vi "21_1.vi"() -> ()   [LabVIEW 2020]
uses:
  <userlib>/_OpenG.lib/array/array.llb/Remove Duplicates from 1D Array (String)__ogtk.vi
  <userlib>/_OpenG.lib/array/array.llb/Index 1D Array Elements (String)__ogtk.vi
panel:
  out "size(s)":i32=1679
  out "Array":string[](array[string])=["tksps", "nmzblnq", "pzz", "gkmdkp", "fdpp", "htdps", "njvzpr", "lsfn", "vxbnd", "qvft", "nmpt", "ptq", "dckbmh", "bh", "xxlb", "pbjp", "zlpbptr", "mmphj", "ddc", "zxmkkpp", "jrgrcz", "xzhmdb", "mqkf", "bmcj", "lsv", "bsbz", "mklt", "nkmj", "crbt", "zxcqtf", "rjbsr", "hbcgjtx", "vvqpqgl", "rnbfzg", "hxndkq", "vrntfjx", "clmk", "zdslsk", "ljczhn", "fkntrq", "kbkkrlfq", "bt", "mrz", "nhpsk", "lsc", "vqjj", "lfd", "bsllxjtm", "zdpcb", "qpjplfl", "gkcskhp", "vrbxt", "ftnhrx", "fbjbkp", "sffzz", "pzvvt", "phth", "mlftm", "kbkkrlfq", "dtqq", "jdnlg", "dlxp", "ljczhn", "zrngn", "qnlrbn", "lbxc", "chjdk", "fkntrq", "xxlb", "pcvh", "xmgc", "vkzh", "pzz", "sgv", "xlc", "xmjr", "bqtpqsp", "vrntfjx", "xxx", "xzhmdb", "vpsd", "clptg", "qpjplfl", "fcrvj", "nmzblnq", "cxgmp", "jqcfq", "sbr", "xbdmll", "jtknrjp", "fcdtf", "bbxvmgs", "mgjdd", "dckbmh", "ns", "fdpp", "pbjp", "xbtpfxjz", "fbvdlb", "mrz", "ftnhrx", "fsddds", "hsmkqgx", "gkmdkp", "xxdmj", "cksrd", "zgbbl", "zdslsk", "zpqbb", "bgkf", "rnbfzg", "bhgzdg", "ndmjr", "nhpsk", "fjndll", "cfnc", "pmqmmxs", "rqpd", "mqkf", "snpxpkvj", "bh", "zbsqdm", "lxkbkkx", "lcpcmk", "xbdmll", "ttszmr", "pzvvt", "jbhhjx", "qfqnpf", "dckbmh", "zgbbl", "vrbxt", "dzbxmn", "bsllxjtm", "dblf", "mlftm", "htdps", "ldprd", "tllqrt", "sfprzmk", "zrngn", "lmxfpn", "hxndkq", "gkcskhp", "bqtpqsp", "chjdk", "kzfsztx", "nkmj", "tjxxdmq", "ztlp", "vvzf", "vplt", "bhgzdg", "gsshb", "bmjx", "fjndll", "clmk", "qbrgtl", "ndmjr", "xzhmdb", "bpzlm", "kspf", "gvhrgz", "ddcrr", "fdpp", "tlgbjhs", "xvqmjsc", "lsc", "mqkf", "lsv", "krrsrp", "zsbzn", "bkxnht", "mgjdd", "jbtjxtf", "slbrp", "kchnq", "vpsd", "zdpcb", "ftnhrx", "sm", "mcdsfh", "xplxv", "fkntrq", "gntk", "tksps", "sbr", "vbxdp", "vtdd", "lrbpxs", "dgnrq", "ktm", "xlc", "jrgrcz", "lkdrpt", "rqpd", "xgzbl", "fjndll", "ddcrr", "xbhsqv", "pqjgdkl", "lxkbkkx", "kttchg", "vvzf", "xxdmj", "xzhmdb", "pbjp", "fcdtf", "kbkkrlfq", "bpzlm", "qlbxr", "ptq", "kzfsztx", "dgnrq", "jbhhjx", "vqjj", "qnlrbn", "kckgz", "cnmm", "zgbbl", "lrbpxs", "ztlp", "hnlcp", "zhlgsj", "bgkf", "zdpcb", "xbtpfxjz", "bsllxjtm", "krrsrp", "pzz", "nhpsk", "mrz", "ndmjr", "zmqvhh", "xxlb", "bqtpqsp", "zsbzn", "qlgb", "ztlp", "gvhrgz", "sfprzmk", "vcvmq", "xxlb", "lmxfpn", "njrdhq", "lcpcmk", "ttszmr", "qbrgtl", "tnzvgg", "hbfmpsg", "hshl", "vvqpqgl", "pzz", "dckbmh", "zlpbptr", "slbrp", "xgxk", "qlbxr", "bmcj", "bqtpqsp", "hsmkqgx", "ftnhrx", "qmxfh", "lbnr", "hbcgjtx", "krrsrp", "nmpt", "fxznf", "zpqbb", "vbxdp", "dtqq", "zdslsk", "mgjdd", "vtdd", "kttchg", "rdtkzbf", "qfqnpf", "ndmjr", "zrngn", "ttszmr", "bqtpqsp", "qvft", "nhpsk", "qfqnpf", "pcvh", "qmxfh", "cksrd", "xxlb", "mcdsfh", "bhgzdg", "nklz", "fcdtf", "mqkf", "pkzjrp", "phth", "zpqbb", "xvqmjsc", "pbjp", "dlxp", "fcrvj", "sfprzmk", "hnlcp", "xbtpfxjz", "hxndkq", "gkmdkp", "vxbnd", "pzz", "clptg", "mlftm", "nmzblnq", "pmqmmxs", "cpjsfp", "cfnc", "xmjr", "nmpt", "sbr", "vvqpqgl", "fxznf", "mcrxr", "hgvszq", "ftnhrx", "vpsd", "vqjj", "bsbz", "pmvs", "gntk", "bt", "kckgz", "fzpcbck", "ddc", "tjxxdmq", "vjpcxq", "prjcx", "pzvvt", "mgjdd", "njrdhq", "xxx", "sffzz", "cksrd", "gvhrgz", "nkmj", "xvqmjsc", "jglfn", "cxgmp", "fkntrq", "vxbnd", "bkdpdr", "ddcrr", "hxndkq", "jclqn", "mrz", "vrntfjx", "fbjbkp", "nmpt", "slbrp", "mcrxr", "tnzvgg", "krrsrp", "jtknrjp", "hsmkqgx", "pmqmmxs", "xxlb", "pbjp", "ndmjr", "xlc", "sbr", "gxnxkkh", "bsd", "kzfsztx", "vvzf", "qmxfh", "jrmj", "tksps", "kchnq", "dgnrq", "nmfd", "mcdsfh", "zmqvhh", "bcv", "qvft", "gsshb", "kspf", "lsfn", "zxmkkpp", "pqjgdkl", "tlgbjhs", "hgvszq", "xbhsqv", "rqpd", "xmgc", "kfghxt", "tjxxdmq", "bmcj", "rjbsr", "fmfj", "zhlgsj", "zsbzn", "xmjr", "ktm", "fcrvj", "pzvvt", "vbxdp", "zpqbb", "pkzjrp", "fcdtf", "ddc", "crbt", "kckgz", "dmrxd", "pmsjc", "nmzblnq", "phth", "qpjplfl", "fsddds", "vplt", "bsbz", "vplt", "nkmj", "bmjx", "vvzf", "rdtkzbf", "qpjplfl", "tlgbjhs", "hsmkqgx", "mgjdd", "bsd", "mklt", "xmjr", "xxdmj", "bkdpdr", "fbjbkp", "ktm", "crbt", "vpsd", "pzz", "fzpcbck", "krrsrp", "zpqbb", "cvrqg", "vcvmq", "xxlb", "vtdd", "htdps", "vvqpqgl", "lsv", "clptg", "kttchg", "jbtjxtf", "ljczhn", "vjpcxq", "dblf", "sfprzmk", "bqtpqsp", "dgnrq", "fcdtf", "dzbxmn", "pzvvt", "chjdk", "jtknrjp", "vf", "ptq", "ddcrr", "lsc", "njvzpr", "jrgrcz", "gkmdkp", "nklz", "lsfn", "ttszmr", "jrmj", "mqkf", "jglfn", "jdnlg", "pmvs", "dtqq", "bsd", "jbtjxtf", "njvzpr", "dblf", "hqvv", "bkxnht", "dzjjxr", "xbtpfxjz", "fxznf", "cvrqg", "qpjplfl", "kspf", "fcdtf", "hbcgjtx", "lsfn", "zhlgsj", "dmrxd", "lsc", "lkdrpt", "nmpt", "dlxp", "hshl", "jclqn", "fkntrq", "sffzz", "lxkbkkx", "lsv", "mcrxr", "mgjdd", "bt", "zxcqtf", "zgbbl", "bh", "pthjxs", "htdps", "pkzjrp", "fbjbkp", "vbxdp", "kbkkrlfq", "pmvs", "pcvh", "zdpcb", "ns", "vrntfjx", "zdpcb", "vbxdp", "jbtjxtf", "zhlgsj", "xbdmll", "qlbxr", "xmjr", "qpjplfl", "pqjgdkl", "gsshb", "fkntrq", "mcdsfh", "ddcrr", "bt", "fbvdlb", "jqcfq", "bgkf", "dtqq", "fmfj", "ddc", "bsllxjtm", "kbkkrlfq", "cpjsfp", "jbhhjx", "qlgb", "vrbxt", "fbjbkp", "gntk", "zrngn", "kckgz", "zlpbptr", "qvft", "hnlcp", "lrbpxs", "bkxnht", "cksrd", "vqjj", "sgv", "dmrxd", "slbrp", "rkzkd", "pthjxs", "cvrqg", "fcrvj", "vtdd", "kchnq", "qbrgtl", "mlftm", "fdpp", "zmqvhh", "jrgrcz", "pzz", "kttchg", "xvqmjsc", "pcvh", "ttszmr", "pzvvt", "bmjx", "gkcskhp", "gvhrgz", "cnmm", "krrsrp", "kbkkrlfq", "gsshb", "vbxdp", "sgv", "kzfsztx", "zbsqdm", "kttchg", "gvhrgz", "rkzkd", "jtknrjp", "hsmkqgx", "rjbsr", "hbcgjtx", "bsllxjtm", "dmrxd", "dzbxmn", "jglfn", "vpsd", "tsnzbdtb", "vcvmq", "xxx", "zlpbptr", "fbjbkp", "lbnr", "hnlcp", "mcrxr", "tllqrt", "lsc", "fjndll", "bbxvmgs", "tksps", "bmjx", "xmjr", "mlftm", "qlgb", "ljczhn", "tjxxdmq", "mrz", "kttchg", "pzz", "xmjr", "vvzf", "ktm", "zhlgsj", "zsbzn", "dckbmh", "vcvmq", "jglfn", "zxmkkpp", "fxznf", "xmgc", "hgvszq", "zlpbptr", "hbfmpsg", "tsnzbdtb", "lkdrpt", "vbxdp", "pqjgdkl", "mlftm", "nhpsk", "ptq", "vjpcxq", "gsshb", "cfnc", "ddcrr", "kckgz", "bh", "kzfsztx", "tnzvgg", "dblf", "xbdmll", "vkzh", "pmqmmxs", "vplt", "nklz", "xplxv", "gvhrgz", "lsfn", "jclqn", "lxkbkkx", "prjcx", "mklt", "hsmkqgx", "vtdd", "sm", "vrntfjx", "rjbsr", "bmcj", "lxkbkkx", "pmqmmxs", "zpqbb", "zmqvhh", "cfnc", "dgnrq", "qpjplfl", "fcdtf", "zsbzn", "zrngn", "vqjj", "nmzblnq", "ldprd", "qvft", "fzpcbck", "xxx", "cpjsfp", "xlc", "clptg", "tksps", "sffzz", "vvzf", "gvhrgz", "jrgrcz", "nhpsk", "lmxfpn", "dzjjxr", "sgv", "tjxxdmq", "pbjp", "jdnlg", "tllqrt", "vxbnd", "htdps", "tlgbjhs", "lfd", "pmsjc", "jglfn", "nmpt", "xbtpfxjz", "vplt", "gntk", "vtdd", "zdslsk", "rqpd", "zdpcb", "vkzh", "clptg", "ldprd", "jglfn", "ztlp", "vrbxt", "vplt", "zbsqdm", "zhlgsj", "crbt", "bcv", "nhpsk", "jbtjxtf", "tllqrt", "xbtpfxjz", "pzvvt", "lkdrpt", "kttchg", "tlgbjhs", "vvzf", "kbkkrlfq", "fbvdlb", "sffzz", "ddcrr", "dlxp", "dckbmh", "gvhrgz", "bgkf", "hxndkq", "lbnr", "slbrp", "bsd", "hsmkqgx", "zpqbb", "gntk", "lcpcmk", "ptq", "gxnxkkh", "nkmj", "vf", "xgxk", "hgvszq", "ns", "jdnlg", "qmxfh", "ddc", "mqkf", "fkntrq", "njrdhq", "gkmdkp", "qmxfh", "bh", "lbnr", "lsc", "xlc", "fzpcbck", "fbvdlb", "njvzpr", "qlgb", "gkmdkp", "xxx", "nhpsk", "bcv", "cpjsfp", "rjbsr", "vvzf", "tsnzbdtb", "lbxc", "ptq", "xvqmjsc", "lrbpxs", "qpjplfl", "rqpd", "tjxxdmq", "ktm", "qlbxr", "sfprzmk", "xgxk", "ldprd", "phth", "fcdtf", "dmrxd", "vtdd", "zmqvhh", "nmfd", "xxlb", "qvft", "mlftm", "bpzlm", "zlpbptr", "fjndll", "vqjj", "zpqbb", "kbkkrlfq", "vf", "gvhrgz", "xplxv", "lsfn", "mmphj", "nmpt", "dzjjxr", "qnlrbn", "tjxxdmq", "slbrp", "chjdk", "kchnq", "ftnhrx", "xxdmj", "gkcskhp", "rkzkd", "mcdsfh", "tlgbjhs", "hgvszq", "bqtpqsp", "bmjx", "ndmjr", "hxndkq", "xxx", "dzbxmn", "htdps", "ldprd", "xmjr", "jclqn", "qbrgtl", "pbjp", "zxcqtf", "zlpbptr", "xlc", "hbfmpsg", "hshl", "lrbpxs", "lsv", "vplt", "vf", "mklt", "tsnzbdtb", "sm", "bcv", "bhgzdg", "pmvs", "fbvdlb", "clptg", "sbr", "pmsjc", "tllqrt", "fkntrq", "kckgz", "fsddds", "lsc", "xbhsqv", "zmqvhh", "bpzlm", "qvft", "fbjbkp", "lcpcmk", "vrntfjx", "mqkf", "vxbnd", "rdtkzbf", "ljczhn", "ptq", "fcrvj", "vpsd", "rkzkd", "qfqnpf", "zrngn", "ftnhrx", "lkdrpt", "qnlrbn", "ljczhn", "hxndkq", "vrntfjx", "xplxv", "lxkbkkx", "bqtpqsp", "tksps", "mgjdd", "pmqmmxs", "crbt", "zgbbl", "dzjjxr", "fsddds", "pzvvt", "lrbpxs", "lcpcmk", "pthjxs", "qlgb", "zmqvhh", "dgnrq", "nhpsk", "lsv", "bkdpdr", "fdpp", "vkzh", "vvzf", "sbr", "vtdd", "nmzblnq", "bt", "zdslsk", "tjxxdmq", "xxlb", "njrdhq", "xbdmll", "clmk", "pcvh", "mcdsfh", "hsmkqgx", "crbt", "lbnr", "jtknrjp", "bt", "nhpsk", "htdps", "hgvszq", "xplxv", "zxcqtf", "cnmm", "jbhhjx", "gkmdkp", "xzhmdb", "ddcrr", "gkcskhp", "pbjp", "fjndll", "xbhsqv", "lmxfpn", "dgnrq", "kttchg", "mcrxr", "sffzz", "vbxdp", "dmrxd", "hbcgjtx", "qlgb", "xbdmll", "dtqq", "bgkf", "cpjsfp", "vpsd", "qpjplfl", "fxznf", "ftnhrx", "jglfn", "dmrxd", "fmfj", "jglfn", "mqkf", "zdslsk", "pmqmmxs", "xmgc", "lxkbkkx", "ndmjr", "dblf", "kckgz", "crbt", "zmqvhh", "dzjjxr", "pkzjrp", "mgjdd", "cpjsfp", "sm", "vxbnd", "kzfsztx", "sffzz", "fbvdlb", "zhlgsj", "gsshb", "fjndll", "hshl", "rjbsr", "lsv", "jqcfq", "jbtjxtf", "bkdpdr", "htdps", "bsd", "mrz", "kttchg", "kbkkrlfq", "xzhmdb", "bhgzdg", "fkntrq", "lmxfpn", "qnlrbn", "bkxnht", "njrdhq", "mklt", "kchnq", "cvrqg", "mcdsfh", "nmfd", "xxlb", "lbnr", "bh", "pzz", "vvqpqgl", "fsddds", "jrmj", "dlxp", "tjxxdmq", "ddc", "vrbxt", "hbfmpsg", "lbxc", "pzvvt", "qlbxr", "sbr", "hnlcp", "rnbfzg", "ttszmr", "fbjbkp", "fzpcbck", "vkzh", "lsfn", "rdtkzbf", "gkcskhp", "fdpp", "sgv", "bpzlm", "vvqpqgl", "rkzkd", "dzbxmn", "phth", "zsbzn", "tllqrt", "bh", "cpjsfp", "lmxfpn", "mgjdd", "fbvdlb", "xzhmdb", "zbsqdm", "nhpsk", "zrngn", "slbrp", "zdslsk", "qnlrbn", "zmqvhh", "xxx", "lxkbkkx", "pqjgdkl", "cvrqg", "jglfn", "vpsd", "lsc", "hsmkqgx", "zdpcb", "gntk", "xbdmll", "dgnrq", "xxdmj", "dckbmh", "ldprd", "rqpd", "bqtpqsp", "xbhsqv", "bcv", "qlgb", "gsshb", "nklz", "lbxc", "sffzz", "ftnhrx", "kfghxt", "nmzblnq", "kttchg", "bmcj", "cnmm", "snpxpkvj", "bgkf", "pmsjc", "zxcqtf", "bhgzdg", "jdnlg", "zgbbl", "fsddds", "ztlp", "fkntrq", "bbxvmgs", "bsbz", "cksrd", "htdps", "jrmj", "lkdrpt", "bqtpqsp", "hshl", "tnzvgg", "zxcqtf", "mklt", "zsbzn", "cfnc", "ns", "clptg", "zhlgsj", "hnlcp", "jtknrjp", "tksps", "vrntfjx", "fbjbkp", "gxnxkkh", "sffzz", "sfprzmk", "bkdpdr", "xmgc", "rjbsr", "lcpcmk", "vjpcxq", "nmpt", "kzfsztx", "qmxfh", "nkmj", "xgzbl", "jqcfq", "bh", "fmfj", "dblf", "sbr", "sm", "gkmdkp", "nklz", "vcvmq", "zdslsk", "xbdmll", "pmvs", "mrz", "xlc", "xxlb", "lbnr", "fjndll", "dzbxmn", "mqkf", "xzhmdb", "nmzblnq", "zdpcb", "nmfd", "lsv", "qlgb", "snpxpkvj", "kchnq", "qfqnpf", "lsfn", "mmphj", "pkzjrp", "vbxdp", "vqjj", "vtdd", "nmzblnq", "lbxc", "zxcqtf", "xplxv", "zdpcb", "lbnr", "qvft", "xbtpfxjz", "bmjx", "zmqvhh", "pzz", "xxdmj", "nkmj", "vvqpqgl", "bsd", "tllqrt", "bpzlm", "lrbpxs", "dtqq", "lmxfpn", "lkdrpt", "fbvdlb", "vcvmq", "cnmm", "dckbmh", "pmqmmxs", "tksps", "njrdhq", "clptg", "ztlp", "chjdk", "tsnzbdtb", "sgv", "htdps", "xmjr", "kckgz", "cxgmp", "dmrxd", "dblf", "vpsd", "rqpd", "rdtkzbf", "sm", "vrntfjx", "bhgzdg", "ktm", "cpjsfp", "ttszmr", "fdpp", "kfghxt", "mmphj", "vvzf", "fjndll", "zxcqtf", "gsshb", "crbt", "dtqq", "cfnc", "bkdpdr", "qlbxr", "fcdtf", "lcpcmk", "zdpcb", "lrbpxs", "hnlcp", "zmqvhh", "snpxpkvj", "vtdd", "qpjplfl", "vrbxt", "nmfd", "pzz", "dlxp", "jrgrcz", "vpsd", "xzhmdb", "bmjx", "lkdrpt", "kzfsztx", "bqtpqsp", "jbhhjx", "pcvh", "fkntrq", "chjdk", "xlc", "jglfn", "fsddds", "tnzvgg", "mrz", "ktm", "hbcgjtx", "lmxfpn", "jbtjxtf", "zgbbl", "ddcrr", "sgv", "zxmkkpp", "kbkkrlfq", "hxndkq", "clmk", "pmqmmxs", "rdtkzbf", "mlftm", "sffzz", "tjxxdmq", "jqcfq", "xgzbl", "qlgb", "zgbbl", "bgkf", "crbt", "pcvh", "clptg", "hnlcp", "fzpcbck", "mqkf", "kzfsztx", "hbfmpsg", "zmqvhh", "zdpcb", "pqjgdkl", "ptq", "mmphj", "pmvs", "vplt", "xbhsqv", "mcdsfh", "rnbfzg", "sfprzmk", "cfnc", "zhlgsj", "jbhhjx", "lfd", "ztlp", "lcpcmk", "lxkbkkx", "cvrqg", "njvzpr", "hbcgjtx", "ktm", "xbtpfxjz", "zlpbptr", "vbxdp", "ljczhn", "nmpt", "fcdtf", "tnzvgg", "qlbxr", "hgvszq", "xgzbl", "xzhmdb", "jrgrcz", "bbxvmgs", "mgjdd", "nklz", "cnmm", "bmjx", "bpzlm", "dmrxd", "dckbmh", "kckgz", "vqjj", "lbxc", "dlxp", "hshl", "nkmj", "fxznf", "fkntrq", "clmk", "bsbz", "xxdmj", "vvqpqgl", "vxbnd", "chjdk", "pzvvt", "vjpcxq", "qvft", "zmqvhh", "dlxp", "zdpcb", "tlgbjhs", "fmfj", "pzz", "ns", "bhgzdg", "vxbnd", "phth", "clmk", "vkzh", "clptg", "xmgc", "lrbpxs", "dckbmh", "bmjx", "fjndll", "mmphj", "fcdtf", "cxgmp", "lfd", "vvzf", "ftnhrx", "ljczhn", "njrdhq", "dtqq", "bkxnht", "zdslsk", "lsv", "bsd", "mlftm", "bqtpqsp", "ndmjr", "mcdsfh", "kttchg", "cpjsfp", "hqvv", "fbvdlb", "pmqmmxs", "sbr", "tnzvgg", "kbkkrlfq", "lkdrpt", "xlc", "xvqmjsc", "fbjbkp", "ldprd", "fzpcbck", "cfnc", "fkntrq", "rdtkzbf", "pmsjc", "xxx", "nhpsk", "jglfn", "zxmkkpp", "nmpt", "hshl", "xmjr", "zpqbb", "fdpp", "vpsd", "pmvs", "lbxc", "tksps", "ddcrr", "fdpp", "zhlgsj", "xbdmll", "xlc", "xvqmjsc", "vxbnd", "fxznf", "clptg", "pzvvt", "crbt", "jbtjxtf", "rjbsr", "ddc", "lmxfpn", "jclqn", "mcdsfh", "xxlb", "nklz", "jrgrcz", "bqtpqsp", "zrngn", "dgnrq", "clmk", "mklt", "ttszmr", "nmzblnq", "xzhmdb", "fkntrq", "zdslsk", "xmgc", "dblf", "ftnhrx", "kspf", "hshl", "dmrxd", "qvft", "dzjjxr", "lxkbkkx", "nmfd", "xgxk", "nhpsk", "vjpcxq", "nkmj", "xplxv", "jglfn", "cxgmp", "zpqbb", "lsc", "tllqrt", "jclqn", "fxznf", "pcvh", "xmgc", "vxbnd", "vvzf", "fsddds", "lmxfpn", "slbrp", "hxndkq", "dmrxd", "snpxpkvj", "tsnzbdtb", "gntk", "phth", "bqtpqsp", "cksrd", "mklt", "lxkbkkx", "tnzvgg", "clptg", "gvhrgz", "mqkf", "rkzkd", "mrz", "hshl", "pthjxs", "bhgzdg", "bkdpdr", "sfprzmk", "bbxvmgs", "clptg", "tllqrt", "xbtpfxjz", "mrz", "clmk", "ktm", "bmjx", "jclqn", "xgxk", "nmzblnq", "bgkf", "kzfsztx", "jrgrcz", "fkntrq", "prjcx", "qbrgtl", "sffzz", "kckgz", "pmqmmxs", "zgbbl", "xxlb", "tlgbjhs", "cvrqg", "rjbsr", "pmvs", "xmgc", "xplxv", "fsddds", "fxznf", "ddc", "fmfj", "qlgb", "xlc", "lfd", "hgvszq", "zmqvhh", "zhlgsj", "fzpcbck", "bhgzdg", "krrsrp", "gxnxkkh", "cksrd", "lxkbkkx", "chjdk", "vrntfjx", "bsd", "gkmdkp", "dblf", "bsllxjtm", "vplt", "mgjdd", "jglfn", "njrdhq", "qfqnpf", "nmfd", "sgv", "vf", "crbt", "cnmm", "bbxvmgs", "nklz", "prjcx", "bmcj", "xxdmj", "cksrd", "pmvs", "vcvmq", "nmfd", "tllqrt", "dckbmh", "nmzblnq", "pkzjrp", "gxnxkkh", "vbxdp", "bh", "jrgrcz", "zhlgsj", "rnbfzg", "ddcrr", "fcrvj", "qlgb", "pmsjc", "mgjdd", "zpqbb", "vrbxt", "zdslsk", "dzjjxr", "qfqnpf", "vpsd", "sffzz", "mklt", "xbdmll", "hbcgjtx", "bt", "xplxv", "jglfn", "kzfsztx", "htdps", "mcrxr", "ldprd", "vvqpqgl", "hnlcp", "kspf", "bpzlm", "qnlrbn", "njrdhq", "fzpcbck", "zsbzn", "xlc", "nklz", "clmk", "dzbxmn", "phth", "fcdtf", "chjdk", "bh", "slbrp", "kttchg", "vkzh", "bsd", "kchnq", "lfd", "bbxvmgs", "cxgmp", "bgkf", "pbjp", "xzhmdb", "hqvv", "rnbfzg", "kzfsztx", "sgv", "hgvszq", "zdslsk", "bkdpdr", "fsddds", "pzvvt", "bmcj", "sbr", "ddcrr", "vbxdp", "cvrqg", "mcrxr", "ldprd", "ljczhn", "sffzz", "pkzjrp", "jclqn", "zmqvhh", "xgxk", "vvqpqgl", "cnmm", "kbkkrlfq", "xbtpfxjz", "hxndkq", "ftnhrx", "crbt", "vcvmq", "nhpsk", "gsshb", "bmjx", "xxlb", "dckbmh", "ns", "lsfn", "bkxnht", "bpzlm", "kfghxt", "xbhsqv", "bsllxjtm", "krrsrp", "qfqnpf", "tlgbjhs", "jbtjxtf", "tksps", "hbcgjtx", "vqjj", "xvqmjsc", "tsnzbdtb", "lrbpxs", "zhlgsj", "fjndll", "bqtpqsp", "bhgzdg", "ttszmr", "hsmkqgx", "jbhhjx", "hshl", "lsc", "mqkf", "jdnlg", "mgjdd", "xxx", "pmvs"]
  in  "Switch":bool
  in  "Input":string="tksps nmzblnq pzz gkmdkp fdpp htdps njvzpr lsfn vxbnd qvft rggkbpj nmpt ptq dckbmh bh xxlb pbjp zlpbptr mmphj ddc zxmkkpp jrgrcz xzhmdb mqkf bmcj nmtzlj dxzq lsv bsbz fvqg mklt dlkxsxg nkmj crbt zxcqtf rjbsr hbcgjtx vvqpqgl rnbfzg hxndkq vrntfjx clmk zdslsk ljczhn fkntrq kbkkrlfq bt mrz nhpsk lsc vqjj gpxmf lfd bsllxjtm zdpcb qpjplfl gkcskhp vrbxt mxf ftnhrx fbjbkp sffzz (contains fish, soy)\npzvvt phth fvqg mlftm gpxmf kbkkrlfq nmtzlj dtqq jdnlg dlxp ljczhn zrngn qnlrbn lbxc chjdk fkntrq xxlb pcvh xmgc vkzh pzz sgv xlc xmjr bqtpqsp vrntfjx xxx dlkxsxg xzhmdb vpsd clptg qpjplfl fcrvj nmzblnq cxgmp jqcfq sbr xbdmll jtknrjp fcdtf bbxvmgs mgjdd dckbmh lmxt dxzq ns fdpp pbjp xbtpfxjz fbvdlb mrz ftnhrx fsddds hsmkqgx gkmdkp xxdmj cksrd zgbbl zdslsk zpqbb bgkf rnbfzg bhgzdg ndmjr nhpsk mxf fjndll cfnc pmqmmxs rqpd mqkf snpxpkvj (contains shellfish)\nbh dxzq zbsqdm lxkbkkx lcpcmk xbdmll ttszmr pzvvt jbhhjx qfqnpf dckbmh zgbbl vrbxt rggkbpj dzbxmn bsllxjtm dblf mlftm fvqg htdps ldprd tllqrt sfprzmk zrngn lmxfpn hxndkq gkcskhp bqtpqsp chjdk kzfsztx nkmj tjxxdmq ztlp dlkxsxg vvzf vplt bhgzdg gsshb lmxt bmjx fjndll clmk qbrgtl ndmjr nmtzlj xzhmdb bpzlm kspf gvhrgz ddcrr fdpp tlgbjhs gpxmf xvqmjsc lsc mqkf lsv krrsrp zsbzn bkxnht mgjdd jbtjxtf slbrp kchnq vpsd zdpcb ftnhrx sm mcdsfh xplxv fkntrq gntk tksps sbr vbxdp vtdd lrbpxs dgnrq ktm (contains sesame, eggs, peanuts)\nxlc dlkxsxg jrgrcz lkdrpt rqpd xgzbl fjndll ddcrr xbhsqv pqjgdkl fvqg mxf lxkbkkx kttchg vvzf xxdmj xzhmdb pbjp fcdtf kbkkrlfq bpzlm qlbxr lmxt rggkbpj ptq kzfsztx dgnrq jbhhjx vqjj qnlrbn kckgz cnmm nmtzlj zgbbl lrbpxs ztlp hnlcp zhlgsj bgkf zdpcb xbtpfxjz bsllxjtm krrsrp pzz nhpsk mrz ndmjr zmqvhh xxlb dxzq bqtpqsp zsbzn (contains dairy, sesame)\nqlgb ztlp gvhrgz sfprzmk vcvmq xxlb lmxfpn njrdhq lcpcmk ttszmr qbrgtl tnzvgg hbfmpsg hshl vvqpqgl pzz dckbmh zlpbptr slbrp xgxk dlkxsxg mxf qlbxr bmcj bqtpqsp hsmkqgx ftnhrx qmxfh fvqg lbnr hbcgjtx krrsrp nmpt fxznf zpqbb lmxt vbxdp dtqq dxzq zdslsk nmtzlj mgjdd gpxmf vtdd kttchg rdtkzbf qfqnpf ndmjr zrngn (contains wheat, fish)\nttszmr bqtpqsp qvft nhpsk qfqnpf pcvh dxzq qmxfh cksrd xxlb mcdsfh bhgzdg nklz fcdtf mqkf pkzjrp phth zpqbb xvqmjsc pbjp dlxp fcrvj sfprzmk hnlcp xbtpfxjz hxndkq gkmdkp vxbnd pzz clptg mlftm nmzblnq pmqmmxs cpjsfp gpxmf cfnc xmjr nmpt sbr vvqpqgl fxznf mcrxr hgvszq ftnhrx dlkxsxg vpsd vqjj bsbz pmvs gntk fvqg bt kckgz fzpcbck ddc tjxxdmq vjpcxq nmtzlj mxf lmxt prjcx pzvvt mgjdd (contains fish)\nnjrdhq xxx sffzz cksrd gvhrgz nkmj xvqmjsc mxf dxzq jglfn cxgmp fkntrq vxbnd bkdpdr ddcrr hxndkq jclqn mrz vrntfjx fbjbkp nmpt slbrp mcrxr tnzvgg krrsrp jtknrjp hsmkqgx gpxmf pmqmmxs xxlb pbjp ndmjr xlc sbr gxnxkkh bsd kzfsztx vvzf qmxfh jrmj tksps kchnq dgnrq nmfd mcdsfh zmqvhh bcv qvft gsshb kspf lsfn zxmkkpp pqjgdkl fvqg tlgbjhs hgvszq nmtzlj xbhsqv rggkbpj rqpd xmgc kfghxt tjxxdmq bmcj rjbsr fmfj zhlgsj zsbzn xmjr ktm fcrvj pzvvt vbxdp zpqbb pkzjrp fcdtf ddc crbt kckgz dmrxd pmsjc lmxt nmzblnq phth qpjplfl fsddds vplt bsbz (contains dairy, wheat)\ndlkxsxg vplt nkmj bmjx vvzf rdtkzbf qpjplfl tlgbjhs hsmkqgx dxzq mgjdd bsd mklt xmjr gpxmf xxdmj bkdpdr fbjbkp fvqg ktm crbt mxf nmtzlj vpsd pzz fzpcbck krrsrp zpqbb cvrqg vcvmq xxlb vtdd htdps vvqpqgl lsv clptg kttchg jbtjxtf ljczhn vjpcxq dblf sfprzmk bqtpqsp dgnrq fcdtf dzbxmn pzvvt chjdk jtknrjp rggkbpj vf ptq ddcrr lsc njvzpr jrgrcz gkmdkp nklz lsfn ttszmr jrmj mqkf jglfn jdnlg pmvs dtqq (contains fish, wheat, shellfish)\nbsd jbtjxtf nmtzlj njvzpr dlkxsxg dblf hqvv bkxnht dzjjxr xbtpfxjz fxznf cvrqg qpjplfl kspf fcdtf hbcgjtx mxf lsfn zhlgsj dmrxd lsc lkdrpt nmpt dlxp hshl jclqn fkntrq sffzz lxkbkkx lsv dxzq mcrxr mgjdd bt zxcqtf zgbbl bh rggkbpj pthjxs htdps gpxmf pkzjrp fbjbkp lmxt vbxdp kbkkrlfq pmvs pcvh zdpcb ns (contains peanuts, fish, dairy)\nvrntfjx dxzq zdpcb vbxdp lmxt jbtjxtf zhlgsj xbdmll qlbxr xmjr qpjplfl pqjgdkl gsshb rggkbpj fkntrq mcdsfh ddcrr bt fbvdlb jqcfq bgkf dtqq fmfj ddc bsllxjtm kbkkrlfq cpjsfp jbhhjx qlgb vrbxt fbjbkp gntk zrngn kckgz nmtzlj zlpbptr qvft hnlcp lrbpxs bkxnht dlkxsxg cksrd vqjj sgv dmrxd slbrp rkzkd pthjxs cvrqg fcrvj vtdd kchnq qbrgtl mlftm mxf fdpp zmqvhh jrgrcz pzz kttchg xvqmjsc pcvh ttszmr fvqg pzvvt bmjx gkcskhp gvhrgz (contains eggs, fish)\ncnmm lmxt krrsrp kbkkrlfq fvqg dlkxsxg gpxmf gsshb vbxdp sgv kzfsztx zbsqdm kttchg gvhrgz rkzkd jtknrjp hsmkqgx rjbsr hbcgjtx bsllxjtm dmrxd dzbxmn jglfn vpsd tsnzbdtb vcvmq xxx zlpbptr fbjbkp lbnr dxzq hnlcp mcrxr rggkbpj tllqrt lsc fjndll bbxvmgs tksps bmjx xmjr mlftm nmtzlj (contains eggs, dairy, shellfish)\nqlgb ljczhn tjxxdmq gpxmf mrz kttchg pzz xmjr vvzf ktm zhlgsj zsbzn dckbmh lmxt nmtzlj vcvmq jglfn zxmkkpp fxznf xmgc hgvszq zlpbptr mxf hbfmpsg tsnzbdtb dxzq lkdrpt vbxdp pqjgdkl mlftm nhpsk ptq vjpcxq gsshb cfnc ddcrr kckgz bh kzfsztx tnzvgg fvqg dblf xbdmll vkzh pmqmmxs dlkxsxg vplt nklz xplxv gvhrgz lsfn jclqn lxkbkkx prjcx mklt hsmkqgx vtdd sm (contains sesame, peanuts, fish)\nvrntfjx rjbsr bmcj lxkbkkx pmqmmxs zpqbb zmqvhh cfnc nmtzlj dgnrq qpjplfl fcdtf zsbzn fvqg zrngn vqjj dlkxsxg nmzblnq ldprd qvft fzpcbck xxx cpjsfp xlc lmxt clptg tksps sffzz vvzf mxf rggkbpj gvhrgz jrgrcz nhpsk lmxfpn dzjjxr sgv tjxxdmq pbjp jdnlg tllqrt vxbnd htdps tlgbjhs lfd gpxmf pmsjc jglfn nmpt xbtpfxjz vplt gntk (contains shellfish, peanuts, fish)\nvtdd zdslsk rqpd zdpcb vkzh clptg ldprd jglfn ztlp mxf vrbxt vplt zbsqdm zhlgsj crbt bcv nhpsk jbtjxtf tllqrt xbtpfxjz pzvvt lkdrpt kttchg tlgbjhs vvzf kbkkrlfq fbvdlb sffzz ddcrr rggkbpj dlxp dckbmh gvhrgz bgkf dxzq fvqg hxndkq lbnr slbrp bsd hsmkqgx zpqbb gntk lcpcmk lmxt ptq gxnxkkh nkmj vf xgxk hgvszq ns jdnlg dlkxsxg qmxfh ddc mqkf fkntrq njrdhq gpxmf gkmdkp (contains shellfish, dairy)\ngpxmf qmxfh bh lbnr fvqg lsc xlc rggkbpj fzpcbck fbvdlb njvzpr qlgb gkmdkp xxx nhpsk bcv nmtzlj cpjsfp lmxt rjbsr vvzf tsnzbdtb lbxc ptq xvqmjsc mxf lrbpxs qpjplfl rqpd tjxxdmq ktm qlbxr sfprzmk dlkxsxg xgxk ldprd phth fcdtf dmrxd vtdd zmqvhh nmfd xxlb qvft mlftm bpzlm zlpbptr fjndll vqjj zpqbb kbkkrlfq vf (contains eggs, fish, soy)\ngvhrgz xplxv lsfn mmphj nmpt dzjjxr qnlrbn tjxxdmq slbrp chjdk kchnq ftnhrx xxdmj gkcskhp rkzkd mcdsfh nmtzlj tlgbjhs hgvszq bqtpqsp bmjx ndmjr hxndkq xxx dzbxmn htdps ldprd xmjr jclqn rggkbpj mxf qbrgtl pbjp zxcqtf zlpbptr xlc hbfmpsg hshl lrbpxs lsv vplt vf mklt gpxmf tsnzbdtb sm bcv lmxt bhgzdg pmvs fbvdlb clptg sbr pmsjc tllqrt fkntrq kckgz fsddds lsc xbhsqv zmqvhh bpzlm qvft fbjbkp lcpcmk vrntfjx fvqg mqkf vxbnd dlkxsxg rdtkzbf ljczhn ptq fcrvj vpsd (contains soy)\nrkzkd qfqnpf zrngn ftnhrx lmxt lkdrpt qnlrbn fvqg ljczhn hxndkq vrntfjx xplxv lxkbkkx bqtpqsp tksps mxf mgjdd pmqmmxs crbt zgbbl dzjjxr fsddds pzvvt lrbpxs lcpcmk pthjxs qlgb gpxmf zmqvhh rggkbpj dgnrq nhpsk lsv bkdpdr fdpp vkzh vvzf dxzq dlkxsxg sbr vtdd nmzblnq bt zdslsk tjxxdmq xxlb njrdhq xbdmll clmk pcvh mcdsfh (contains shellfish, dairy)\nhsmkqgx crbt lbnr jtknrjp bt nhpsk htdps hgvszq xplxv zxcqtf cnmm jbhhjx gkmdkp nmtzlj xzhmdb ddcrr gkcskhp pbjp fjndll xbhsqv lmxfpn dgnrq kttchg dxzq mcrxr sffzz vbxdp dmrxd hbcgjtx fvqg qlgb xbdmll mxf dtqq rggkbpj bgkf gpxmf cpjsfp vpsd lmxt qpjplfl fxznf ftnhrx jglfn (contains peanuts, wheat, sesame)\ndmrxd fmfj jglfn mqkf zdslsk pmqmmxs xmgc lxkbkkx ndmjr dblf kckgz crbt zmqvhh dzjjxr pkzjrp nmtzlj mgjdd fvqg cpjsfp sm vxbnd kzfsztx sffzz fbvdlb zhlgsj gsshb fjndll hshl rjbsr lsv jqcfq jbtjxtf bkdpdr htdps bsd mrz kttchg kbkkrlfq xzhmdb bhgzdg fkntrq lmxfpn qnlrbn bkxnht njrdhq mklt kchnq cvrqg mcdsfh nmfd xxlb lbnr bh pzz dxzq vvqpqgl fsddds mxf jrmj dlxp lmxt tjxxdmq gpxmf ddc vrbxt hbfmpsg lbxc pzvvt qlbxr sbr hnlcp rnbfzg ttszmr fbjbkp fzpcbck dlkxsxg vkzh lsfn rdtkzbf gkcskhp fdpp (contains shellfish, peanuts, dairy)\nsgv bpzlm vvqpqgl rkzkd dzbxmn phth zsbzn tllqrt bh cpjsfp lmxfpn dlkxsxg mgjdd fbvdlb xzhmdb zbsqdm nhpsk zrngn slbrp zdslsk qnlrbn zmqvhh xxx lxkbkkx pqjgdkl cvrqg jglfn vpsd lsc dxzq hsmkqgx mxf zdpcb gntk xbdmll dgnrq xxdmj dckbmh ldprd rqpd bqtpqsp fvqg gpxmf rggkbpj xbhsqv bcv qlgb gsshb nklz lbxc sffzz lmxt ftnhrx kfghxt nmzblnq kttchg bmcj cnmm snpxpkvj bgkf pmsjc zxcqtf bhgzdg jdnlg zgbbl fsddds ztlp fkntrq (contains wheat, eggs)\nbbxvmgs dlkxsxg bsbz cksrd htdps jrmj fvqg lkdrpt bqtpqsp hshl tnzvgg zxcqtf mklt zsbzn cfnc ns clptg zhlgsj hnlcp jtknrjp tksps vrntfjx fbjbkp gxnxkkh lmxt sffzz rggkbpj sfprzmk bkdpdr xmgc rjbsr lcpcmk vjpcxq nmpt kzfsztx qmxfh nkmj xgzbl jqcfq bh fmfj dblf mxf gpxmf sbr sm gkmdkp nklz vcvmq zdslsk dxzq xbdmll pmvs mrz xlc xxlb lbnr fjndll dzbxmn mqkf xzhmdb nmzblnq zdpcb nmfd lsv qlgb snpxpkvj kchnq qfqnpf lsfn mmphj pkzjrp vbxdp (contains fish)\nvqjj vtdd nmzblnq lbxc zxcqtf xplxv zdpcb lbnr qvft xbtpfxjz bmjx dlkxsxg zmqvhh pzz xxdmj nkmj vvqpqgl bsd tllqrt bpzlm lrbpxs dtqq fvqg lmxfpn lkdrpt fbvdlb vcvmq cnmm dckbmh pmqmmxs tksps njrdhq clptg rggkbpj gpxmf ztlp chjdk tsnzbdtb sgv htdps xmjr kckgz cxgmp dmrxd dblf vpsd rqpd rdtkzbf nmtzlj sm vrntfjx bhgzdg lmxt dxzq ktm cpjsfp ttszmr fdpp kfghxt (contains soy)\nmmphj vvzf fjndll zxcqtf gsshb crbt dtqq cfnc bkdpdr qlbxr fcdtf mxf lcpcmk zdpcb lrbpxs hnlcp zmqvhh snpxpkvj vtdd qpjplfl rggkbpj vrbxt nmfd pzz dlxp jrgrcz vpsd xzhmdb bmjx lkdrpt kzfsztx bqtpqsp jbhhjx pcvh fkntrq chjdk xlc jglfn fsddds tnzvgg mrz ktm gpxmf hbcgjtx lmxfpn jbtjxtf dxzq fvqg zgbbl dlkxsxg ddcrr sgv zxmkkpp kbkkrlfq hxndkq clmk pmqmmxs rdtkzbf mlftm lmxt sffzz tjxxdmq jqcfq xgzbl (contains peanuts)\nqlgb rggkbpj zgbbl lmxt bgkf nmtzlj crbt pcvh clptg hnlcp fzpcbck mqkf kzfsztx hbfmpsg zmqvhh zdpcb pqjgdkl ptq mmphj pmvs vplt xbhsqv mcdsfh rnbfzg sfprzmk cfnc zhlgsj fvqg jbhhjx lfd ztlp lcpcmk lxkbkkx cvrqg njvzpr hbcgjtx ktm mxf xbtpfxjz zlpbptr vbxdp ljczhn nmpt fcdtf tnzvgg qlbxr gpxmf hgvszq xgzbl xzhmdb jrgrcz bbxvmgs mgjdd nklz cnmm bmjx bpzlm dmrxd dckbmh kckgz vqjj lbxc dlxp hshl nkmj fxznf fkntrq clmk bsbz xxdmj vvqpqgl vxbnd chjdk pzvvt dlkxsxg vjpcxq (contains dairy, peanuts)\nqvft zmqvhh gpxmf dlxp zdpcb tlgbjhs fmfj pzz ns bhgzdg vxbnd phth clmk vkzh clptg rggkbpj xmgc lrbpxs dckbmh bmjx fjndll mmphj fcdtf cxgmp lfd vvzf ftnhrx ljczhn lmxt njrdhq dtqq bkxnht zdslsk lsv bsd mlftm bqtpqsp ndmjr mcdsfh kttchg cpjsfp hqvv fbvdlb pmqmmxs sbr tnzvgg kbkkrlfq lkdrpt xlc nmtzlj xvqmjsc fbjbkp ldprd fzpcbck cfnc fkntrq mxf rdtkzbf pmsjc xxx nhpsk jglfn zxmkkpp nmpt hshl xmjr dlkxsxg fvqg zpqbb fdpp vpsd pmvs (contains shellfish, peanuts, fish)\nlbxc tksps mxf ddcrr nmtzlj fdpp zhlgsj xbdmll xlc xvqmjsc vxbnd fxznf clptg pzvvt crbt jbtjxtf rjbsr ddc lmxfpn jclqn mcdsfh xxlb nklz jrgrcz dlkxsxg bqtpqsp zrngn dgnrq clmk mklt ttszmr nmzblnq xzhmdb fkntrq zdslsk xmgc dblf ftnhrx kspf rggkbpj hshl lmxt fvqg dmrxd qvft dzjjxr lxkbkkx nmfd xgxk nhpsk gpxmf vjpcxq (contains soy, sesame, fish)\nnkmj xplxv fvqg jglfn cxgmp zpqbb lsc tllqrt jclqn fxznf lmxt rggkbpj dlkxsxg pcvh xmgc vxbnd vvzf fsddds lmxfpn slbrp hxndkq gpxmf dmrxd snpxpkvj tsnzbdtb gntk phth bqtpqsp cksrd nmtzlj mklt lxkbkkx tnzvgg clptg gvhrgz mqkf rkzkd mrz hshl pthjxs bhgzdg bkdpdr sfprzmk mxf bbxvmgs (contains soy, shellfish)\nclptg tllqrt xbtpfxjz mrz clmk ktm bmjx jclqn xgxk gpxmf nmzblnq lmxt bgkf kzfsztx jrgrcz fkntrq prjcx qbrgtl sffzz kckgz pmqmmxs zgbbl mxf xxlb tlgbjhs cvrqg rjbsr rggkbpj dxzq pmvs xmgc xplxv fsddds fxznf ddc fmfj qlgb xlc lfd hgvszq zmqvhh zhlgsj fzpcbck bhgzdg krrsrp gxnxkkh cksrd lxkbkkx chjdk vrntfjx bsd gkmdkp dblf bsllxjtm nmtzlj vplt mgjdd jglfn njrdhq qfqnpf nmfd sgv vf crbt dlkxsxg (contains wheat, sesame)\ncnmm bbxvmgs nklz prjcx bmcj xxdmj cksrd pmvs vcvmq nmfd tllqrt dckbmh nmzblnq pkzjrp gxnxkkh vbxdp bh lmxt jrgrcz zhlgsj gpxmf rnbfzg ddcrr fcrvj qlgb pmsjc mgjdd zpqbb mxf vrbxt zdslsk dzjjxr qfqnpf vpsd sffzz mklt xbdmll hbcgjtx bt xplxv jglfn kzfsztx dlkxsxg fvqg htdps mcrxr dxzq ldprd nmtzlj vvqpqgl hnlcp kspf bpzlm qnlrbn (contains sesame, soy, fish)\nnjrdhq fzpcbck zsbzn xlc nklz clmk dzbxmn phth nmtzlj dxzq fcdtf chjdk bh slbrp kttchg vkzh bsd gpxmf kchnq lfd bbxvmgs cxgmp bgkf pbjp dlkxsxg xzhmdb hqvv rnbfzg kzfsztx sgv hgvszq zdslsk bkdpdr fsddds pzvvt bmcj sbr mxf ddcrr vbxdp cvrqg mcrxr ldprd ljczhn sffzz pkzjrp jclqn zmqvhh xgxk rggkbpj vvqpqgl cnmm kbkkrlfq xbtpfxjz hxndkq ftnhrx crbt vcvmq nhpsk gsshb bmjx xxlb dckbmh ns lsfn bkxnht bpzlm kfghxt xbhsqv bsllxjtm krrsrp qfqnpf tlgbjhs jbtjxtf tksps hbcgjtx vqjj xvqmjsc tsnzbdtb lrbpxs zhlgsj fjndll bqtpqsp bhgzdg ttszmr hsmkqgx jbhhjx hshl lsc mqkf lmxt jdnlg mgjdd xxx pmvs (contains shellfish, wheat)"
  in  "Input Test":string="mxmxvkd kfcds sqjhc nhms (contains dairy, fish)\ntrh fvjkl sbzzf mxmxvkd (contains dairy)\nsqjhc fvjkl (contains soy)\nsqjhc mxmxvkd sbzzf (contains fish)"
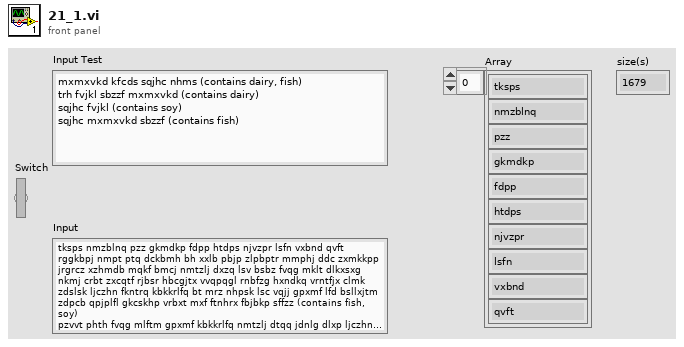
[diagram p1: front panel]
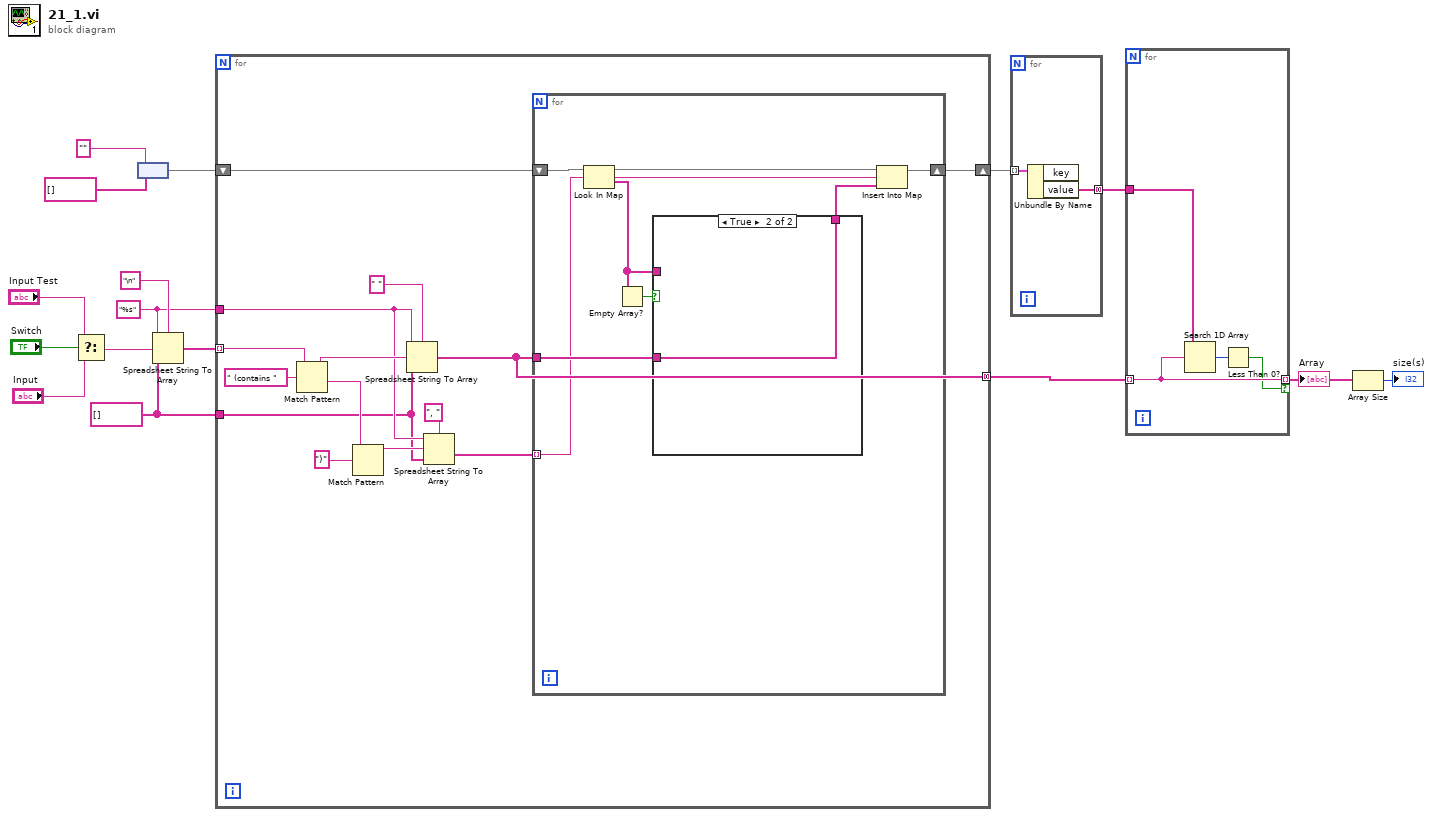
[diagram p0: block diagram]
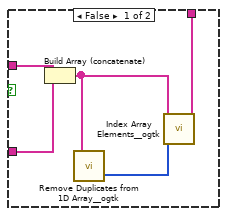
[diagram p2: hidden frame]
diagram:
  w6 = string[] []
  w7 = "%s"
  n1 = Select(t="Input Test", s="Switch", f="Input") -> (s? t:f=w13:string)
  n2 = node("", string[] []) -> (w8:map{string, string[]})
  n3 = Spreadsheet String To Array(delimiter (Tab)="\n", format string=w7, spreadsheet string=w13, array type (2D Dbl)=w6) -> (array=w11:string[])
  n4 = for {
    tunnel: w11 -> [w30] mode=indexing
    shift-right: [w19] -> w5
    shift-left: w8 -> [w20]
    tunnel: w7 -> [w22]
    tunnel: w6 -> [w21]
    tunnel: [w17] -> w3 mode=concatenating
    n5 = Match Pattern(string=w30, regular expression=" (contains ") -> (before substring=w28:string, after substring=w26:string)  [unwired: 1 in, 2 out]
    n6 = Match Pattern(string=w26, regular expression=")") -> (before substring=w24:string)  [unwired: 1 in, 3 out]
    n7 = Spreadsheet String To Array(delimiter (Tab)=" ", format string=w22, spreadsheet string=w28, array type (2D Dbl)=w21) -> (array=w17:string[])
    n8 = Spreadsheet String To Array(delimiter (Tab)=", ", format string=w22, spreadsheet string=w24, array type (2D Dbl)=w21) -> (array=w18:string[])
    n9 = for {
      shift-right: [w36] -> w19
      shift-left: w20 -> [w37]
      tunnel: w17 -> [w35]
      tunnel: w18 -> [w33] mode=indexing
      n10 = Look In Map(map=w37, key=w33) -> (value=w32:string[])  [unwired: 1 in, 1 out]
      n11 = Empty Array?(array=w32) -> (empty?=w31:bool)
      n12 = case shown="True" w31 {
        tunnel: w35 -> [w41 w43]
        tunnel: [w39 w43] -> w34
        tunnel: w32 -> [w38 _]
        frame False {
          n13 = Build Array (concatenate)(w38, w41) -> (w40:string[])
          n14 = call-poly <userlib>:"Remove Duplicates from 1D Array__ogtk.vi"("Input Array"=w40) -> ("indices of removed elements"=w42:i32[])  [unwired: 1 out]
          n15 = call-poly <userlib>:"Index Array Elements__ogtk.vi"("indices"=w42, "array"=w40) -> ("elements"=w39:string[])  [unwired: 9 in]
        }
        frame True {
        }
      }
      n16 = Insert Into Map(map in=w37, key=w33, value=w34) -> (map out=w36:map{string, string[]})  [unwired: 2 out]
    }
  }
  n17 = for {
    tunnel: w5 -> [w45] mode=indexing
    tunnel: [w44] -> w4 mode=concatenating
    n18 = Unbundle By Name(w45) -> ("value"=w44:string[])  [unwired: 1 out]
  }
  n19 = for {
    tunnel: w3 -> [w48] mode=indexing
    tunnel: w4 -> [w49]
    tunnel: [w48] -> w2 mode=indexing if=w46
    n20 = Search 1D Array(1D array=w49, element=w48) -> (index of element=w47:i32)  [unwired: 1 in]
    n21 = Less Than 0?(x=w47) -> (x < 0?=w46:bool)
  }
  "Array" <- w2
  n22 = Array Size(array=w2) -> (size(s)=→"size(s)":i32)
